vi "subCleanUpDependencies.vi"(8 "error in (no error)":errorcluster, 11 "SolutionBuilder in":refnum<class "SolutionBuilder.lvclass">) -> (0 "error out":errorcluster, 3 "SolutionBuilder out":refnum<class "SolutionBuilder.lvclass">)   [LabVIEW 2020, in "SolutionBuilder.lvlib" / "SolutionBuilder.lvclass"]
uses:
  SolutionBuilder.lvclass
  SolutionBuilder.lvclass/SolutionBuilder.ctl
  ProjectItem/ProjectItem.lvclass
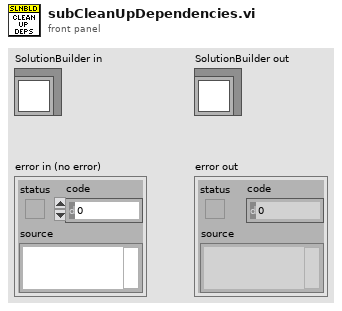
[diagram p1: front panel]
types:
  T1 = typedef "SolutionBuilder.lvlib/SolutionBuilder.lvclass/ProjectItemMap.ctl" = map{path, refnum<class "ProjectItem.lvclass">[]}
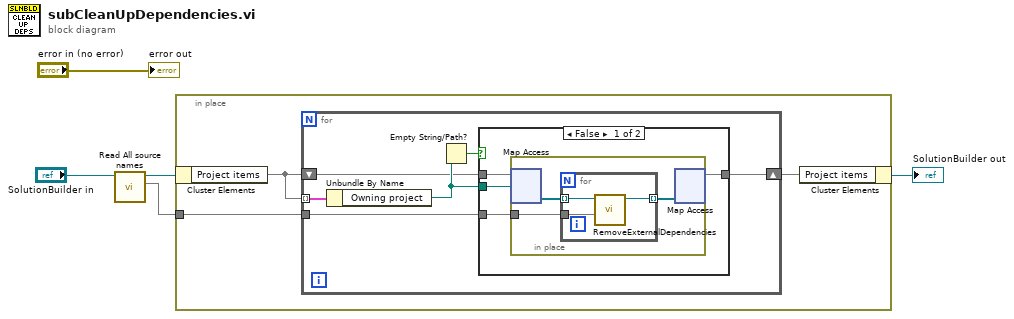
[diagram p0: block diagram]
diagram:
  n1 = call-dynamic "Read All source names.vi"("SolutionBuilder in"="SolutionBuilder in") -> ("All source names"=w2:set{string}, "SolutionBuilder out"=w3:refnum<class "SolutionBuilder.lvclass">)  [unwired: 9 in]
  n2 = in-place {
    in-place-border: w2 -> [w7]
    n3 = in-place-cluster #1(w3) -> ("Project items"=w8:T1)
    n4 = for {
      tunnel: w8 -> [w14] mode=indexing
      shift-right: [w9] -> w6
      shift-left: w8 -> [w11]
      tunnel: w7 -> [w10]
      n5 = Unbundle By Name(w14) -> ("Owning project"=w12:path)
      n6 = Empty String/Path?(string/path=w12) -> (empty?=w13:bool)
      n7 = case shown="False" w13 {
        tunnel: w12 -> [w17 _]
        tunnel: w11 -> [w18 w25]
        tunnel: w10 -> [w16 _]
        tunnel: [w15 w25] -> w9
        frame False {
          n8 = in-place {
            in-place-border: w16 -> [w20]
            n9 = in-place-map #2(w18, w17) -> (w21:refnum<class "ProjectItem.lvclass">[])  [unwired: 1 in, 1 out]
            n10 = for {
              tunnel: w21 -> [w24] mode=indexing
              tunnel: w20 -> [w23]
              tunnel: [w22] -> w19 mode=indexing
              n11 = call-dynamic "RemoveExternalDependencies.vi"("Possible deps"=w23, "ProjectItem in"=w24) -> ("ProjectItem out"=w22:refnum<class "ProjectItem.lvclass">)  [unwired: 8 in, 1 out]
            }
            n12 = in-place-map #2(w19) -> (w15:T1)  [unwired: 1 in, 2 out]
          }
        }
        frame True {
        }
      }
    }
    n13 = in-place-cluster #1("Project items"=w6) -> (→"SolutionBuilder out":refnum<class "SolutionBuilder.lvclass">)
  }
  "error out" <- "error in (no error)"
